vi "Initiate Timeout.vi"(7 "Timeout Period in ms (-1, never)":i32=-1, 8 "error in (no error)":errorcluster, 9 "Target in":refnum<class "State.lvclass">, 10 "Context in":refnum<class "Context.lvclass">, 11 "Source in":refnum<class "State.lvclass">) -> (0 "error out":errorcluster, 1 "Target out":refnum<class "State.lvclass">, 2 "Context out":refnum<class "Context.lvclass">, 3 "Source out":refnum<class "State.lvclass">)   [LabVIEW 2024, in "State.lvlib" / "State.lvclass"]
uses:
  State.lvclass
  Context/Context/Context.lvclass
  State.lvclass/State.ctl
  <vilib>/ActorFramework/Time-Delayed Send Message/Time-Delay Override Options.ctl
  State Machine Messages/Timeout Msg/Timeout Msg.lvclass
  C:/Program Files (x86)/National Instruments/LabVIEW 2024/vi.lib/ActorFramework/Message/Message.lvclass
  <vilib>/ActorFramework/Message Enqueuer/Message Enqueuer.lvclass
  C:/Users/ottoa/OneDrive/Desktop/working copies/stateMachineActor/src/State Machine/State Machine Messages/Timeout Msg/Timeout Msg.lvclass
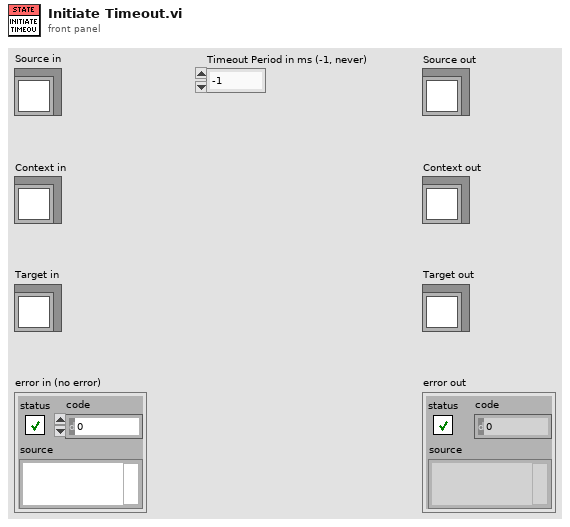
[diagram p1: front panel]
types:
  T1 = typedef "Time-Delay Override Options.ctl" = enum16{"Send next copy now", "Skip next scheduled copy", "Send next copy now and stop all further copies", "Stop all further copies"}
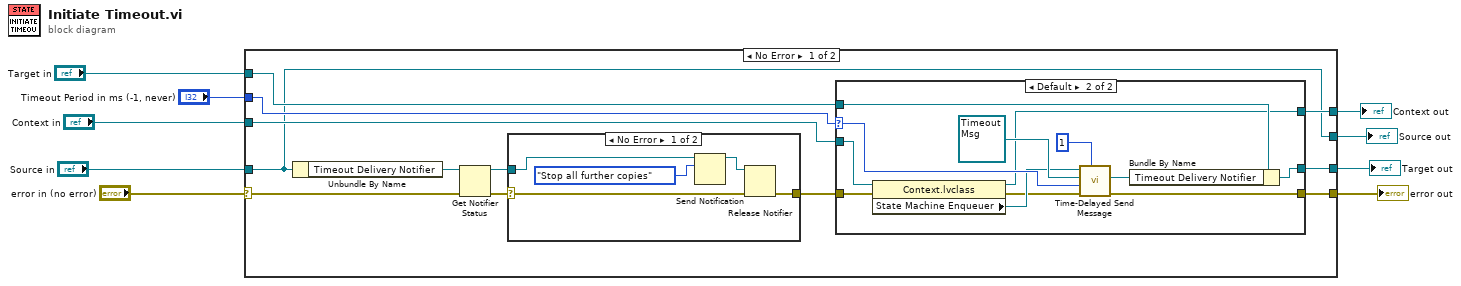
[diagram p0: block diagram]
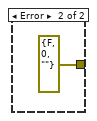
[diagram p2: hidden frame]
diagram:
  n1 = case shown="No Error" "error in (no error)" {
    selector: "error in (no error)" -> [w13 w46]
    tunnel: [w12 w46] -> w8
    tunnel: [w14 w44] -> w6
    tunnel: "Source in" -> [w10 w43]
    tunnel: "Timeout Period in ms (-1, never)" -> [w17 _]
    tunnel: "Context in" -> [w16 w45]
    tunnel: [w15 w45] -> w3
    tunnel: "Target in" -> [w11 w44]
    tunnel: [w10 w43] -> w1
    frame No Error {
      n2 = Unbundle By Name(w10) -> ("Timeout Delivery Notifier"=w20:refnum<notifier>)
      n3 = Get Notifier Status(notifier=w20, error in (no error)=w13) -> (notifier out=w18:refnum<notifier>, error out=w19:errorcluster)  [unwired: 3 out]
      n4 = case shown="No Error" w19 {
        selector: w19 -> [w26 _]
        tunnel: [w25 errorcluster {"status"=FALSE, "code"=0, "source"=""} ("error out")] -> w21
        tunnel: w18 -> [w22 _]
        frame No Error {
          n5 = Send Notification(notification=Time-Delay_Override_Options."Stop all further copies", notifier=w22) -> (notifier out=w23:refnum<notifier>)  [unwired: 1 in, 1 out]
          n6 = Release Notifier(notifier=w23, error in (no error)=w26) -> (error out=w25:errorcluster)  [unwired: 1 in, 2 out]
        }
        frame Error {
        }
      }
      n7 = case shown="Default" w17 {
        selector: w17 -> [_ w40]
        tunnel: [w30 w37] -> w14
        tunnel: w11 -> [w30 w39]
        tunnel: w21 -> [w28 w32]
        tunnel: [w28 w36] -> w12
        tunnel: w16 -> [w29 w35]
        tunnel: [w29 w34] -> w15
        frame -1 {
        }
        frame Default {
          n8 = property class="Context.lvclass"(reference=w35, error in=w32) -> (reference out=w34:refnum<class "Context.lvclass">, error out=w31:errorcluster, "State Machine Enqueuer"=w33:refnum<class "Message Enqueuer.lvclass">)
          n9 = call <vilib>:"Time-Delayed Send Message.vi"("# Copies (0 = infinite repeat)"=u32 1, "error in (no error)"=w31, "Milliseconds To Wait"=w40, "Message"=refnum<class "Timeout Msg.lvclass"> refnum ("State Machine.lvlib:Timeout Msg.lvclass"), "Message Enqueuer"=w33) -> ("error out"=w36:errorcluster, "Delivery Notifier"=w38:refnum<notifier>)  [unwired: 5 in]
          n10 = Bundle By Name(cluster=w39, "Timeout Delivery Notifier"=w38) -> (w37:refnum<class "State.lvclass">)
        }
      }
    }
    frame Error {
    }
  }
  "error out" <- w8
  "Target out" <- w6
  "Context out" <- w3
  "Source out" <- w1
